vi "Mask Write Holding Register1.vi"(4 "OR mask":u16, 6 "AND mask":u16, 7 "Unit_ID":T1, 8 "error in (no error)":errorcluster, 10 "address":u16, 11 "Modbus master in":refnum<class "TCP.lvclass">) -> (0 "error out":errorcluster, 3 "Modbus master out":refnum<class "TCP.lvclass">)   [LabVIEW 2019, in "NI_modbus_upd.lvlib"]
doc: "Writes values to one or more bits of a holding register."
uses:
  TCP/TCP.lvclass
  Ctl/Unit_ID.ctl
  TCP/TCP.lvclass/TCP.ctl
  Function code mismatch error1.vi
  Error Generator1.vi
  Modbus Data Unit (PDU)/Construct PDU1.vi
  Read ADU Packet Master.vi
  Write ADU Packet Master.vi
  Modbus Data Unit (PDU)/Unflatten to PDU1.vi
  TCP/Protocol Read.vi
  TCP/Protocol Write.vi
  <vilib>/Utility/error.llb/Error Cluster From Error Code.vi
  Modbus Data Unit (PDU)/Deconstruct PDU1.vi
  NI_modbus_upd.lvlib
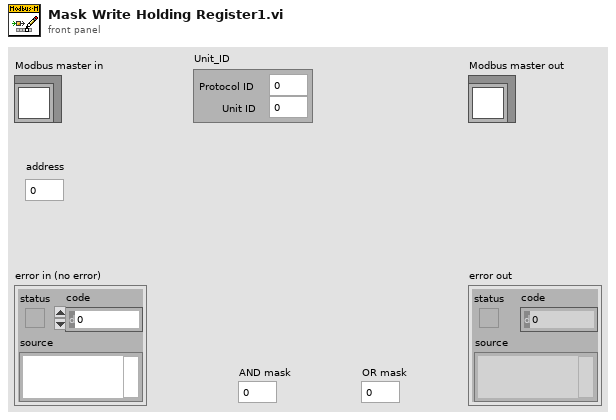
[diagram p1: front panel]
types:
  T1 = typedef "NI_modbus_upd.lvlib/Unit_ID.ctl" = cluster{"Protocol ID":u16, "Unit ID":u8}
  T2 = typedef "NI_modbus_upd.lvlib/MB Modbus Data Unit.ctl" = cluster{"function":T3, "Data":u8[]}
  T3 = typedef "NI_modbus_upd.lvlib/Function.ctl" = u8
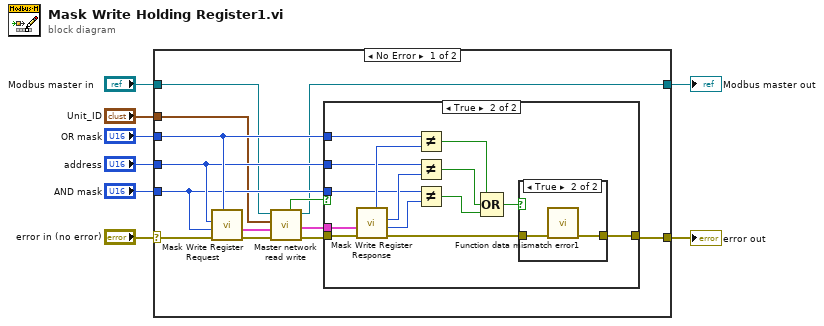
[diagram p0: block diagram]
diagram:
  n1 = case shown="No Error" "error in (no error)" {
    selector: "error in (no error)" -> [w10 w40]
    tunnel: "Modbus master in" -> [w12 w41]
    tunnel: [w14 w41] -> w7
    tunnel: [w20 w40] -> w6
    tunnel: "OR mask" -> [w18 _]
    tunnel: "address" -> [w17 _]
    tunnel: "AND mask" -> [w16 _]
    tunnel: "Unit_ID" -> [w9 _]
    frame No Error {
      n2 = call "Mask Write Register Request.vi"("OR mask"=w18, "error in (no error)"=w10, "AND mask"=w16, "starting address"=w17) -> ("error out"=w21:errorcluster, "Modbus Data Unit out"=w13:T2)  [unwired: 6 in]
      n3 = call "Master network read write.vi"("error in (no error)"=w21, "Modbus Data Unit"=w13, "Unit_ID"=w9, "TCP in"=w12) -> ("error out"=w19:errorcluster, "Modbus data unit out"=w11:T2, "TCP out"=w14:refnum<class "TCP.lvclass">, "PDU valid?"=w15:bool)  [unwired: 4 in]
      n4 = case shown="True" w15 {
        tunnel: [w22 w34] -> w20
        tunnel: w19 -> [w22 w31]
        tunnel: w18 -> [_ w26]
        tunnel: w16 -> [_ w25]
        tunnel: w17 -> [_ w24]
        tunnel: w11 -> [_ w23]
        frame False {
        }
        frame True {
          n5 = call "Mask Write Register Response.vi"("error in (no error)"=w31, "Modbus Data Unit in"=w23) -> ("error out"=w30:errorcluster, "AND mask"=w32:u16, "address"=w33:u16, "OR mask"=w27:u16)  [unwired: 6 in]
          n6 = Not Equal?(x=w26, y=w27) -> (x != y?=w28:bool)
          n7 = Not Equal?(x=w24, y=w33) -> (x != y?=w29:bool)
          n8 = Not Equal?(x=w25, y=w32) -> (x != y?=w36:bool)
          n9 = Compound Arithmetic op=OR(w28, w29, w36) -> (w35:bool)
          n10 = case shown="True" w35 {
            tunnel: [w37 w39] -> w34
            tunnel: w30 -> [w37 w38]
            frame False {
            }
            frame True {
              n11 = call "Function data mismatch error1.vi"("error in (no error)"=w38) -> ("error out"=w39:errorcluster)  [unwired: 10 in]
            }
          }
        }
      }
    }
    frame Error {
    }
  }
  "error out" <- w6
  "Modbus master out" <- w7
